vi "Escritura en Base de Datos.vi"() -> ()   [LabVIEW 2020]
uses:
  <vilib>/httpClient/PUTBuffer.vi
  <vilib>/httpClient/LabVIEWHTTPClient.lvlib
panel:
  in  "stop 2":bool
  in  "Dial":dbl(knob) scale=0.0..10.0
  in  "Led rele":bool
  out "body PUT":string
  out "headers PUT":string
  out "error PUT":errorcluster
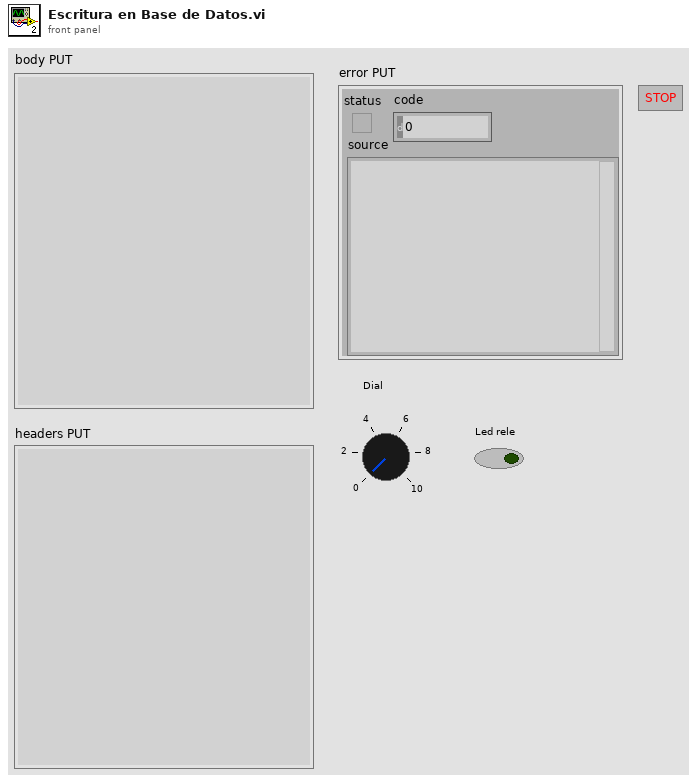
[diagram p1: front panel]
types:
  T1 = cluster{"Acondicionamiento":dbl, "Data":string, "Hora":string, "Led rele":bool}
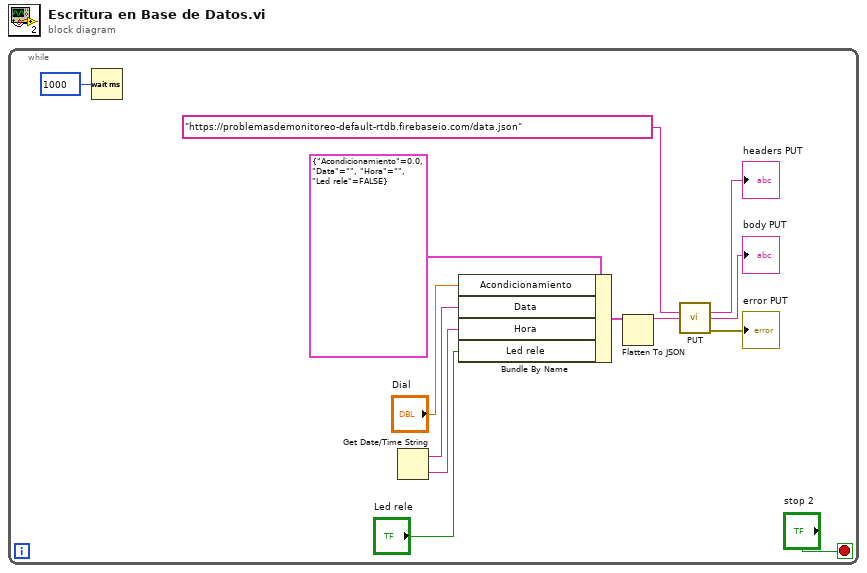
[diagram p0: block diagram]
diagram:
  n1 = while {
    stop <- "stop 2" stop-if-true
    n2 = Wait (ms)(milliseconds to wait=u32 1000) -> ()  [unwired: 1 out]
    n3 = Get Date/Time String() -> (date string=w9:string, time string=w8:string)  [unwired: 3 in]
    n4 = Bundle By Name(cluster=T1 {"Acondicionamiento"=0.0, "Data"="", "Hora"="", "Led rele"=FALSE}, "Acondicionamiento"="Dial", "Data"=w9, "Hora"=w8, "Led rele"="Led rele") -> (w7:T1)
    n5 = Flatten To JSON(anything=w7) -> (JSON string=w5:string)  [unwired: 2 in, 1 out]
    n6 = call-poly <vilib>:"PUT.vi"("url"="https://problemasdemonitoreo-default-rtdb.firebaseio.com/data.json", "buffer"=w5) -> ("headers"=→"headers PUT":string, "body"=→"body PUT":string, "error out"=→"error PUT":errorcluster)  [unwired: 10 in, 1 out]
  }
